vi "PC_AIChar_v2.vi"() -> ()   [LabVIEW 2019]
uses:
  TypeDefs/UIStateDefEnum.ctl
  <vilib>/measure/maspectr.llb/Power Spectrum and PSD Export Mode.ctl
  <vilib>/Analysis/baseanly.llb/Mean (DBL).vi
  <vilib>/Analysis/5stat.llb/RMS (DBL).vi
  <vilib>/NI/STM/TCP/Read Meta Data (TCP Ref).vi
  <vilib>/NI/STM/TCP/Get Connection Reference (TCP).vi
  <vilib>/measure/maspectr.llb/FFT Power Spectrum and PSD for 1 Chan.vi
  <vilib>/NI/STM/TCP/Read Meta Data (TCP Clst).vi
  <vilib>/NI/STM/TCP/Read Message (TCP).vi
  <vilib>/NI/STM/NI STM.lvlib
  <vilib>/Analysis/NI_AALBase.lvlib
  <vilib>/measure/NI_MAPro.lvlib
  <vilib>/Analysis/NI_AALPro.lvlib
  Components/Spectra/Spectra.lvlib
panel:
  in  "Select\nTarget":enum16{"myRIO", "cRIO"}(ring)
  out "Analysis Loop \ntime [s]":dbl format="%#.4g"
  out "Analysis \ntime-span [s]":dbl format="%.2f"
  out "# of elements \nremoved":i32
  in  "Pause Charts":bool
  in  "Clear charts":bool
  out "RT target \nloop \ntime [s]":dbl=0.0002
  out "Data length \n[count]":i32
  out "Mean [V]":dbl format="%#.6f"
  out "RMS / \nStd. Dev. [mV]":dbl format="%#.6f"
  out "Spectra plots":cluster{"f0":dbl, "df":dbl, "magnitude":dbl[]}[](graph)
  out "Histogram Graph":T1(graph)
  out "STM Loop \ntime [s]":dbl format="%#.4g"
  in  "System Stop Button":bool
  out "Data":dbl[][](graph)
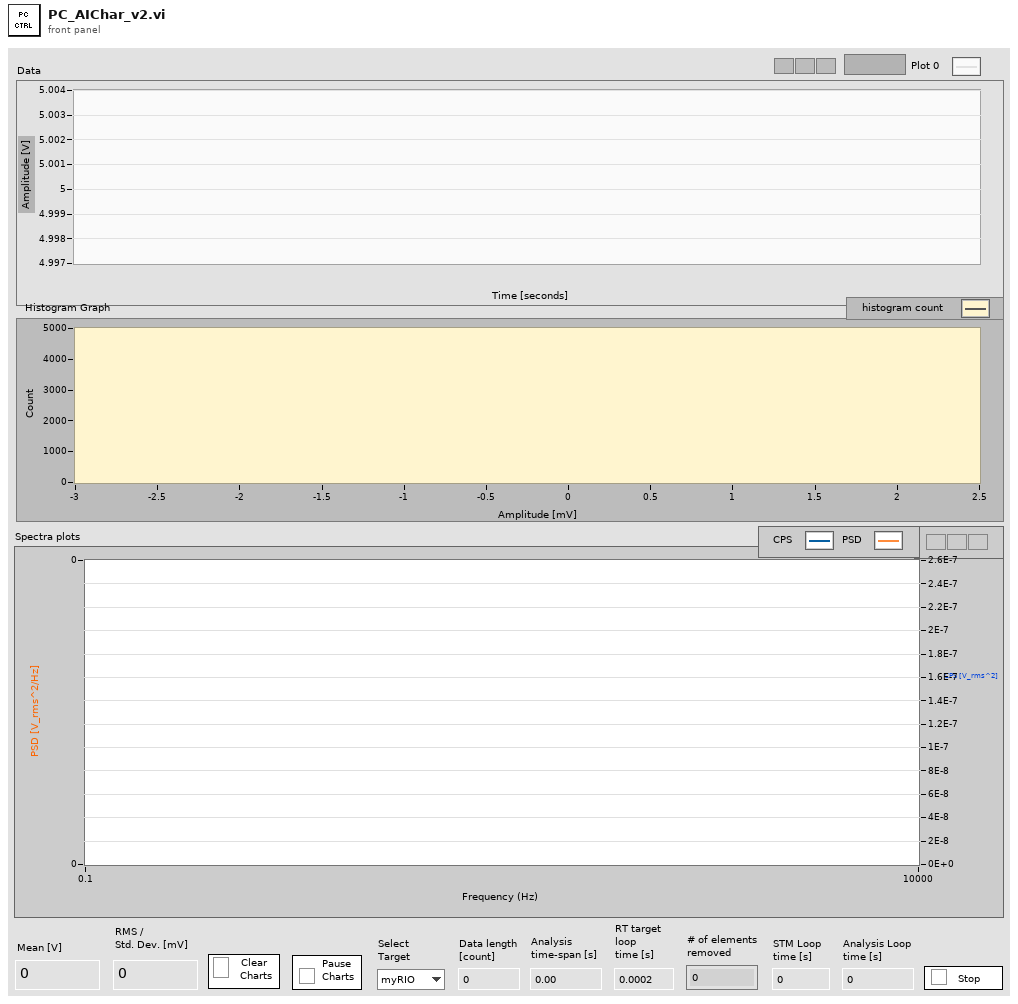
[diagram p1: front panel]
types:
  T1 = cluster{"X Values":dbl[], "Histogram: h(x)":i32[]}
  T2 = typedef "UIStateDefEnum.ctl" = enum16{"Wait", "Initialize", "Clear", "Stop"}
  T3 = typedef "NI STM.lvlib/TCP Connection Info.ctl" = cluster{"connection ID":refnum<k5>, "meta data":T4[]}
  T4 = typedef "NI STM.lvlib/MetaDataElement.ctl" = string
  T5 = typedef "NI_MAPro.lvlib/Power Spectrum and PSD Export Mode.ctl" = u16
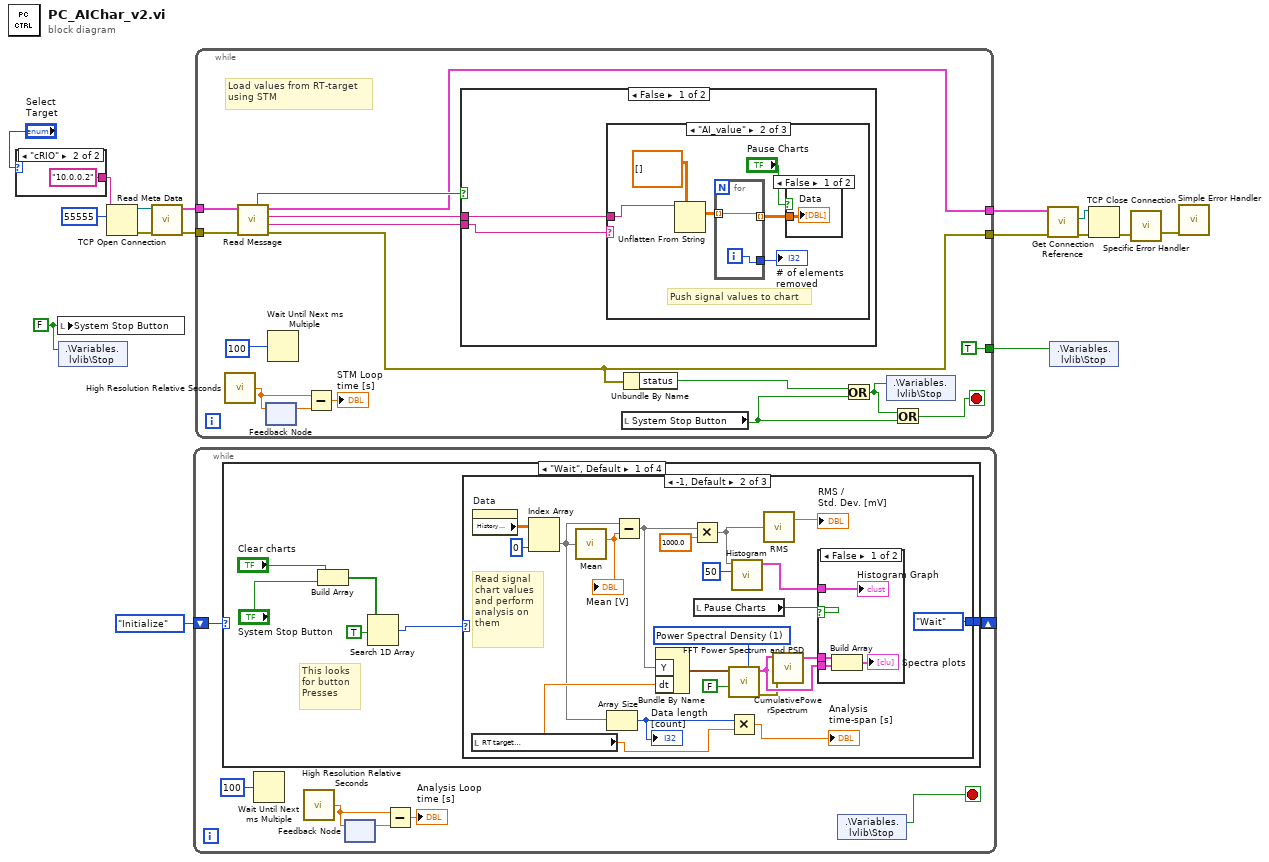
[diagram p0: block diagram]
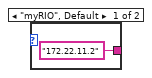
[diagram p2: hidden frame]
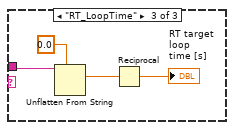
[diagram p5: hidden frame]
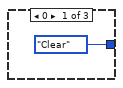
[diagram p7: hidden frame]
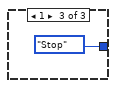
[diagram p9: hidden frame]
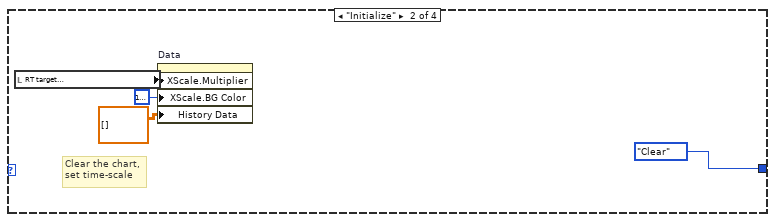
[diagram p10: hidden frame]
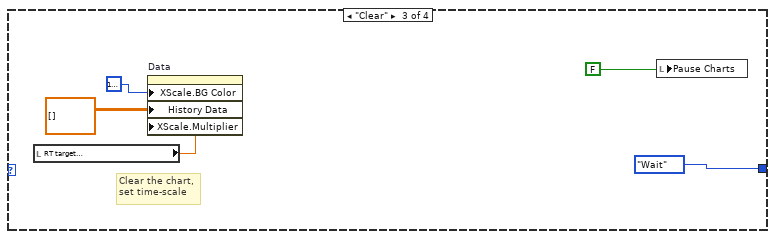
[diagram p11: hidden frame]
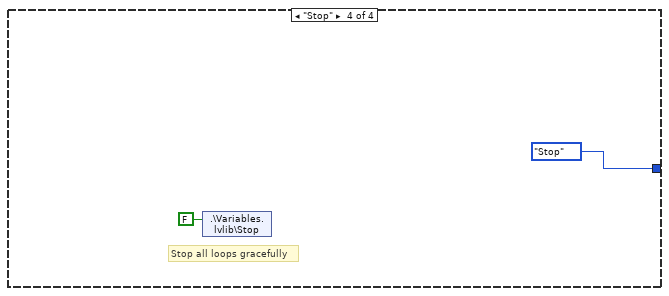
[diagram p12: hidden frame]
diagram:
  w4 = FALSE ("System Stop Button")
  n1 = case shown="\"cRIO\"" "Select\nTarget" {
    tunnel: ["172.22.11.2" ("address") "10.0.0.2" ("address")] -> w15
    frame "myRIO", Default {
    }
    frame "cRIO" {
    }
  }
  n2 = local write "System Stop Button"(w4) -> ()
  n3 = shared-variable ".\\Variables.lvlib\\Stop"(w4) -> ()  [unwired: 1 in, 1 out]
  n4 = TCP Open Connection(address=w15, remote port or service name=u16 55555) -> (connection ID=w14:refnum<k5>, error out=w13:errorcluster)  [unwired: 3 in]
  n5 = call-poly <vilib>:"Read Meta Data.vi"("error in"=w13, "connection ID"=w14) -> ("error out"=w11:errorcluster, "connection info out"=w12:T3)  [unwired: 7 in, 1 out]
  n6 = while {
    shift-right: [w23] -> _
    shift-left: UIStateDefEnum."Initialize" ("UIStateDefEnum") -> [w24]
    stop <- w22 stop-if-true
    n7 = case shown="\"Wait\", Default" w24 {
      tunnel: [w26 UIStateDefEnum."Clear" ("UIStateDefEnum") UIStateDefEnum."Wait" ("UIStateDefEnum") UIStateDefEnum."Stop" ("UIStateDefEnum")] -> w23
      frame "Wait", Default {
        # "This looks \nfor button \nPresses"
        n8 = Build Array "Build Array"("Clear charts", "System Stop Button") -> (w31:bool[])
        n9 = Search 1D Array(1D array=w31, element=TRUE) -> (index of element=w27:i32)  [unwired: 1 in]
        n10 = case shown="-1, Default" w27 {
          tunnel: [UIStateDefEnum."Clear" ("UIStateDefEnum") UIStateDefEnum."Wait" ("UIStateDefEnum") UIStateDefEnum."Stop" ("UIStateDefEnum")] -> w26
          frame 0 {
          }
          frame -1, Default {
            w49 = T5 1 items=["Power Spectrum", "Power Spectral Density"] ("export mode")
            # "Read signal\nchart values\nand perform\nanalysis on \nthem"
            n11 = local read "RT target \nloop \ntime [s]"() -> (w42:dbl)
            n12 = property on="Data" class="WFChart (strict)"() -> ("History Data"=w47:dbl[][])  [unwired: 2 in, 2 out]
            n13 = Index Array(array=w47, index (col)=0 ("disabled index (col)")) -> (element=w37:dbl[])  [unwired: 1 in]
            n14 = call-poly <vilib>:"Mean.vi"("X"=w37) -> ("mean"=w48:dbl)  [unwired: 1 out]
            "Mean [V]" <- w48
            n15 = Array Size(array=w37) -> (size(s)=w43:i32)
            "Data length \n[count]" <- w43
            n16 = Subtract(x=w37, y=w48) -> (x-y=w36:dbl[])
            n17 = Bundle By Name("Y"=w36, "dt"=w42) -> (w51:waveform(dbl))  [unwired: 1 in]
            n18 = Multiply(x=w36, y=1000.0) -> (x*y=w38:dbl[])
            n19 = local read "Pause Charts"() -> (w41:bool)
            n20 = call-poly <vilib>:"FFT Power Spectrum and PSD.vi"("export mode"=w49, "dB On (F)"=FALSE, "time signal"=w51) -> ("error out"=w33:errorcluster, "Power Spectrum / PSD"=w34:cluster{"f0":dbl, "df":dbl, "magnitude":dbl[]})  [unwired: 5 in, 2 out]
            n21 = Multiply(x=w43, y=w42) -> (x*y=→"Analysis \ntime-span [s]":dbl)
            n22 = call <vilib>:"Histogram.vi"("intervals"=50, "X"=w38) -> ("Histogram Graph"=w52:T1)  [unwired: 6 in, 3 out]
            n23 = call-poly <vilib>:"RMS.vi"("X"=w38) -> ("rms value"=→"RMS / \nStd. Dev. [mV]":dbl)  [unwired: 1 out]
            n24 = call "CumulativePowerSpectrum.vi"("error in (no error)"=w33, "PSD"=w34) -> ("CPS"=w35:cluster{"f0":dbl, "df":dbl, "magnitude":dbl[]})  [unwired: 8 in, 1 out]
            n25 = case shown="False" w41 {
              tunnel: w52 -> [w57 _]
              tunnel: w35 -> [w56 _]
              tunnel: w34 -> [w54 _]
              frame False {
                n26 = Build Array(w56, w54) -> (→"Spectra plots":cluster{"f0":dbl, "df":dbl, "magnitude":dbl[]}[])
                "Histogram Graph" <- w57
              }
              frame True {
              }
            }
          }
          frame 1 {
          }
        }
      }
      frame "Initialize" {
        # "Clear the chart,\nset time-scale"
        n27 = local read "RT target \nloop \ntime [s]"() -> (w61:dbl)
        n28 = property on="Data" class="WFChart (strict)"("XScale.Multiplier"=w61, "XScale.BG Color"=u32 16777216 ("X Scale.Marker Colors:BG Color"), "History Data"=dbl[][] []) -> ()  [unwired: 2 in, 2 out]
      }
      frame "Clear" {
        # "Clear the chart,\nset time-scale"
        n29 = local read "RT target \nloop \ntime [s]"() -> (w63:dbl)
        n30 = property on="Data" class="WFChart (strict)"("XScale.BG Color"=u32 16777216 ("X Scale.Marker Colors:BG Color"), "History Data"=dbl[][] [], "XScale.Multiplier"=w63) -> ()  [unwired: 2 in, 2 out]
        n31 = local write "Pause Charts"(FALSE ("Pause Charts")) -> ()
      }
      frame "Stop" {
        # "Stop all loops gracefully"
        n32 = shared-variable ".\\Variables.lvlib\\Stop"(FALSE ("Stop")) -> ()  [unwired: 1 in, 1 out]
      }
    }
    n33 = Wait Until Next ms Multiple(millisecond multiple=u32 100) -> ()  [unwired: 1 out]
    n34 = call <vilib>:"High Resolution Relative Seconds.vi"() -> ("relative seconds"=w20:dbl)
    n35 = feedback #1() -> (w21:dbl)  [unwired: 1 in]
    n36 = feedback-in #1(w20) -> ()
    n37 = Subtract(x=w20, y=w21) -> (x-y=→"Analysis Loop \ntime [s]":dbl)
    n38 = shared-variable ".\\Variables.lvlib\\Stop"() -> (w22:bool)  [unwired: 1 in, 1 out]
  }
  n39 = while {
    tunnel: w12 -> [w85]
    tunnel: w11 -> [w84]
    tunnel: [w82] -> w7
    tunnel: [w81] -> w6
    tunnel: [TRUE ("Stop")] -> w2
    stop <- w75 stop-if-true
    # "Load values from RT-target\nusing STM"
    n40 = call <vilib>:"High Resolution Relative Seconds.vi"() -> ("relative seconds"=w77:dbl)
    n41 = call-poly <vilib>:"Read Message.vi"("error in"=w84, "connection info in"=w85) -> ("error out"=w81:errorcluster, "name"=w80:T4, "data string"=w79:string, "connection info out"=w82:T3, "timed out?"=w83:bool)  [unwired: 4 in, 1 out]
    n42 = feedback-in #2(w77) -> ()
    n43 = feedback #2() -> (w78:dbl)  [unwired: 1 in]
    n44 = Wait Until Next ms Multiple(millisecond multiple=u32 100 ("Period")) -> ()  [unwired: 1 out]
    n45 = Subtract(x=w77, y=w78) -> (x-y=→"STM Loop \ntime [s]":dbl)
    n46 = case shown="False" w83 {
      tunnel: w80 -> [w87 _]
      tunnel: w79 -> [w86 _]
      frame False {
        n47 = case shown="\"AI_value\"" w87 {
          tunnel: w86 -> [_ w92 w97]
          frame Default {
          }
          frame "AI_value" {
            # "Push signal values to chart"
            n48 = Unflatten From String(type=dbl[][] [], binary string=w92) -> (value=w91:dbl[][])  [unwired: 3 in, 2 out]
            n49 = for {
              tunnel: w91 -> [w96] mode=indexing
              tunnel: [w96] -> w90 mode=indexing
              tunnel: [w95] -> w89
              i -> [w95]
            }
            "# of elements \nremoved" <- w89
            n50 = case shown="False" "Pause Charts" {
              tunnel: w90 -> [w94 _]
              frame False {
                "Data" <- w94
              }
              frame True {
              }
            }
          }
          frame "RT_LoopTime" {
            n51 = Unflatten From String(type=0.0, binary string=w97) -> (value=w99:dbl)  [unwired: 3 in, 2 out]
            n52 = Reciprocal(x=w99) -> (1/x=→"RT target \nloop \ntime [s]":dbl)
          }
        }
      }
      frame True {
      }
    }
    n53 = local read "System Stop Button"() -> (w74:bool)
    n54 = Unbundle By Name(w81) -> ("status"=w73:bool)
    n55 = Or(x=w73, y=w74) -> (x .or. y?=w72:bool)
    n56 = shared-variable ".\\Variables.lvlib\\Stop"(w72) -> ()  [unwired: 1 in, 1 out]
    n57 = Or(x=w72, y=w74) -> (x .or. y?=w75:bool)
  }
  n58 = call-poly <vilib>:"Get Connection Reference.vi"("error in"=w6, "connection info in"=w7) -> ("error out"=w10:errorcluster, "connection ID out"=w9:refnum<k5>)  [unwired: 7 in, 1 out]
  n59 = shared-variable ".\\Variables.lvlib\\Stop"(w2) -> ()  [unwired: 1 in, 1 out]
  n60 = TCP Close Connection(connection ID=w9, error in (no error)=w10) -> (error out=w8:errorcluster)  [unwired: 1 in, 1 out]
  n61 = call "Specific Error Handler"("Error to Check"=w8) -> ("error out"=w5:errorcluster)  [unwired: 11 in, 3 out]
  n62 = call <vilib>:"Simple Error Handler.vi"("error in (no error)"=w5) -> ()  [unwired: 4 in, 5 out]
